vi "Initialize Item.vi"(7 "Item Type":T1, 8 "error in (no error)":errorcluster, 11 "Path":path) -> (0 "error out":errorcluster, 3 "Item":refnum<class "Item.lvclass">)   [LabVIEW 2020, in "VI Properties Editor.lvlib"]
uses:
  VI Properties Editor.lvlib
  Item/Item.lvclass
  VI/VI.lvclass
  C:/Users/User/Documents/LabVIEW Data/Projects/VI-Properties-Editor/source/Classes/Item/Item.lvclass
  C:/Users/User/Documents/LabVIEW Data/Projects/VI-Properties-Editor/source/Classes/VI/VI.lvclass
  Item Type.ctl
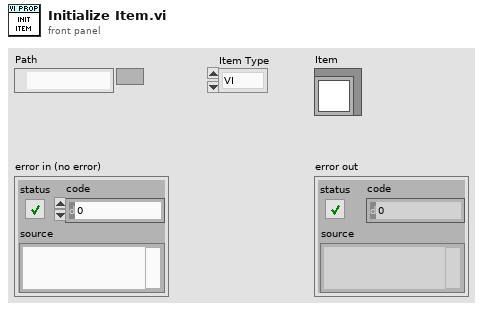
[diagram p1: front panel]
types:
  T1 = typedef "VI Properties Editor.lvlib/Item Type.ctl" = enum16{"VI"}
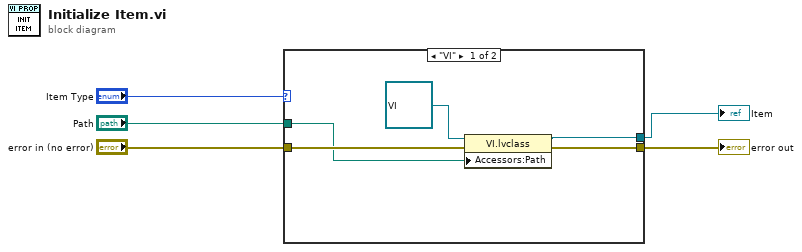
[diagram p0: block diagram]
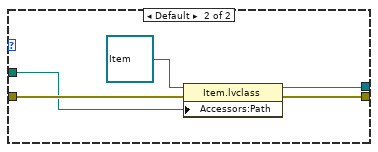
[diagram p2: hidden frame]
diagram:
  n1 = case shown="\"VI\"" "Item Type" {
    tunnel: "error in (no error)" -> [w9 w15]
    tunnel: "Path" -> [w8 w14]
    tunnel: [w7 w13] -> w2
    tunnel: [w6 w11] -> w1
    frame "VI" {
      n2 = property class="VI.lvclass"(reference=refnum<class "VI.lvclass"> refnum ("VI Properties Editor.lvlib:VI.lvclass"), error in=w9, "Accessors:Path"=w8) -> (reference out=w6:refnum<class "VI.lvclass">, error out=w7:errorcluster)
    }
    frame Default {
      n3 = property class="Item.lvclass"(reference=refnum<class "Item.lvclass"> refnum ("VI Properties Editor.lvlib:Item.lvclass"), error in=w15, "Accessors:Path"=w14) -> (reference out=w11:refnum<class "Item.lvclass">, error out=w13:errorcluster)
    }
  }
  "error out" <- w2
  "Item" <- w1
